vi "Make_Different_Variants_of_Tracks-6.vi"(8 "error IN":errorcluster, 9 "[IN] # of Longest track\nInside the Group of Tracks":i32, 10 "[IN] Index of Earliest \nProblem Point Inside":i32, 11 "[IN] Still connected\ntracks in group":T2) -> (0 "error OUT":errorcluster, 1 "[OUT] Index of # tracks \nwith problem points":i32[](array[numeric]), 2 "[OUT] Index of connected \npoints inside the track":i32[](array[numeric]), 3 "[OUT] Subtracks":T1(array[cluster]), 4 "[OUT] Status of 1st Problem Point":i16, 5 "[OUT] 2 or more subtracks":bool)   [LabVIEW 2017]
doc: "The subVI formates competing subtracks \nTwo cases are considered: \nSplitting event => only variants after splitting + account the origin of one of subtracks\nMerging event => competition between different variants of elongations"
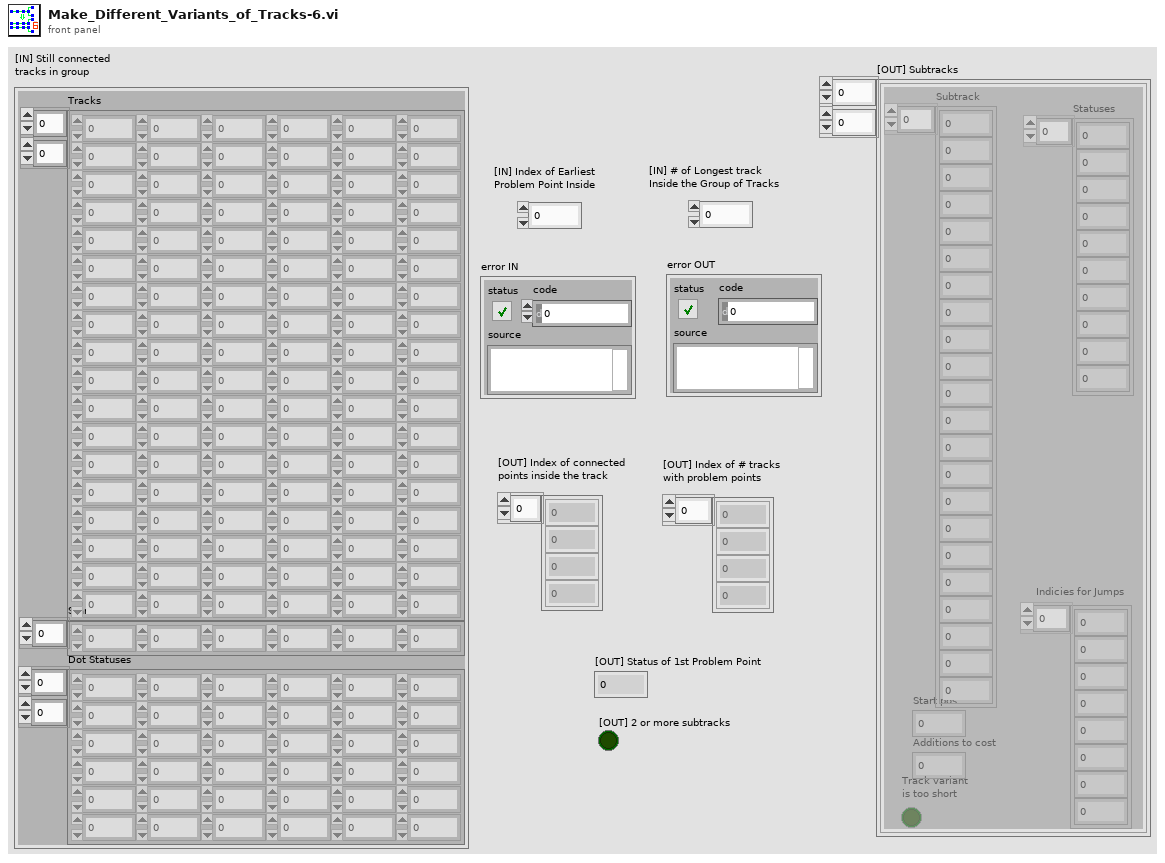
[diagram p1: front panel]
types:
  T1 = cluster{"Subtrack":dbl[], "Statuses":i16[], "Start pos":i32, "Additions to cost":i8, "Track variant \nis too short":bool, "Indicies for Jumps":i32[]}[][]
  T2 = cluster{"Tracks":dbl[][], "Start Pos":i32[], "Dot Statuses":i16[][]}
  T3 = cluster{"Subtrack":dbl[], "Statuses":i16[], "Start pos":i32, "Additions to cost":i8, "Track variant \nis too short":bool, "Indicies for Jumps":i32[]}
  T4 = cluster{"Subtrack":dbl[], "Statuses":i16[], "Start pos":i32, "Additions to cost":i8, "Track variant \nis too short":bool, "Indicies for Jumps":i32[]}[]
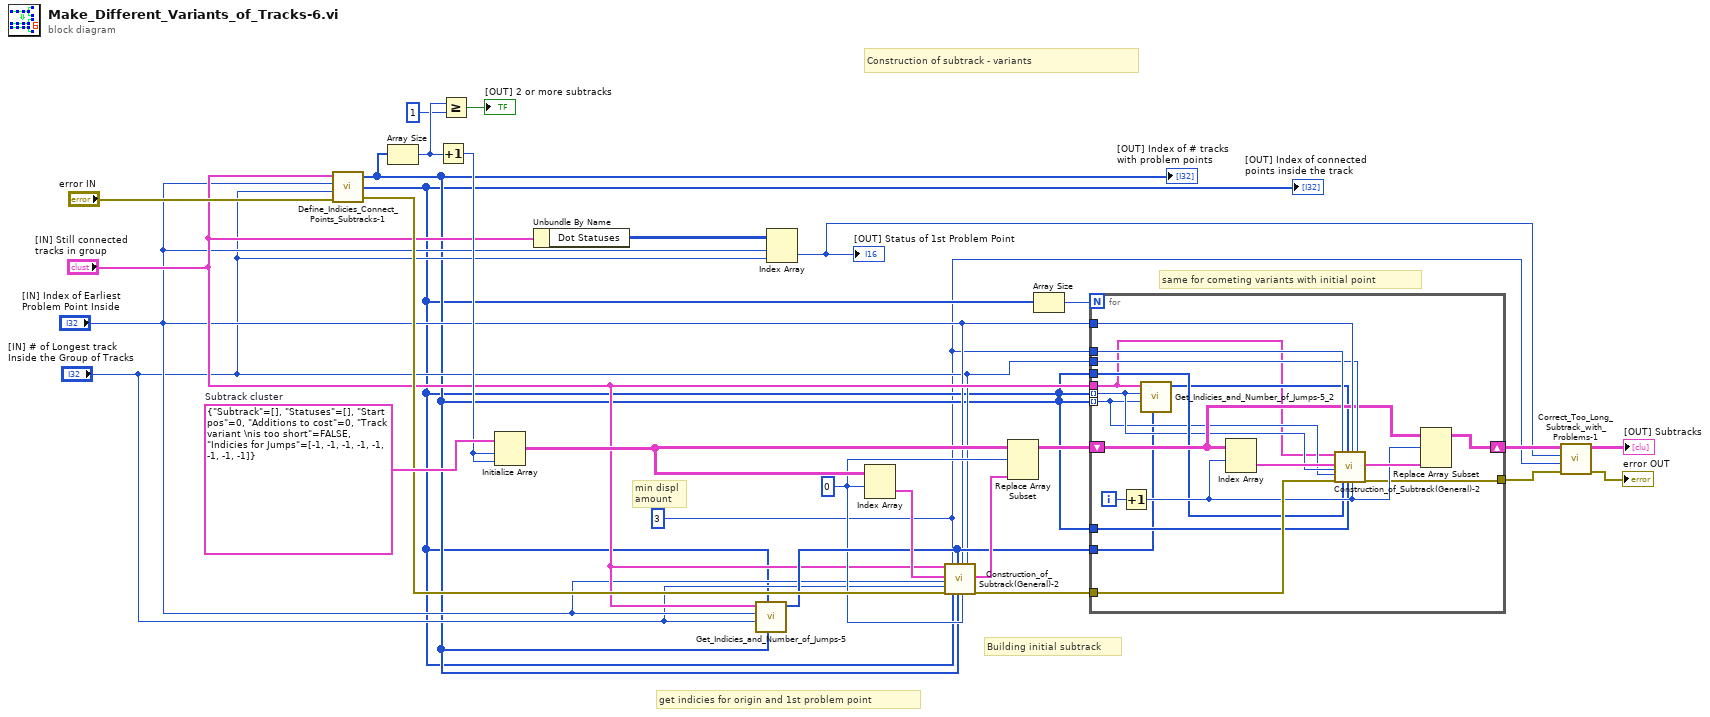
[diagram p0: block diagram]
diagram:
  w16 = 0
  w1 = 3 ("[IN] Minimal Subtrack Length \n(Points without problems) for\nMaking Desicion")
  w27 = T3 {"Subtrack"=[], "Statuses"=[], "Start pos"=0, "Additions to cost"=0, "Track variant \nis too short"=FALSE, "Indicies for Jumps"=[-1, -1, -1, -1, -1, -1, -1, -1]}  # Subtrack cluster
  # "same for cometing variants with initial point"
  # "Building initial subtrack"
  # "get indicies for origin and 1st problem point"
  # "min displ \namount"
  # "Construction of subtrack - variants"
  n1 = call "Define_Indicies_Connect_Points_Subtracks-1.vi"("error IN"="error IN", "[IN] Index of track with\n(problem displacement)"="[IN] # of Longest track\nInside the Group of Tracks", "[IN] Index of problem\ndisplacement inside track"="[IN] Index of Earliest \nProblem Point Inside", "[IN] Track group"="[IN] Still connected\ntracks in group") -> ("error OUT"=w18:errorcluster, "[OUT] Index of \nconnected dots\ninside the track"=w10:i32[], "[OUT] Index of connected\ntracks with problem dot"=w11:i32[])
  "[OUT] Index of connected \npoints inside the track" <- w10
  "[OUT] Index of # tracks \nwith problem points" <- w11
  n2 = Array Size(array=w11) -> (size(s)=w9:i32)
  n3 = Increment(x=w9) -> (x+1=w23:i32)
  n4 = Greater Or Equal?(x=w9, y=1) -> (x >= y?=→"[OUT] 2 or more subtracks":bool)
  n5 = Initialize Array(w27, w23, w23) -> (w26:T1)
  n6 = Unbundle By Name("[IN] Still connected\ntracks in group") -> ("Dot Statuses"=w14:i16[][])
  n7 = call "Get_Indicies_and_Number_of_Jumps-5.vi"("[IN] Index of connected\ntracks with problem dot"=w11, "[IN] Index of connected \ndots inside the track"=w10, "[IN] # of Track with\nFirst Problem Point"="[IN] # of Longest track\nInside the Group of Tracks", "[IN] Index of First Pro\nblem Point Inside Track"="[IN] Index of Earliest \nProblem Point Inside", "[IN] Still connected\ntracks in group"="[IN] Still connected\ntracks in group") -> ("[OUT] Indicies for Jumps"=w17:i32[])  [unwired: 5 in]
  n8 = Index Array(array=w14, index (row)="[IN] Index of Earliest \nProblem Point Inside", index (col)="[IN] # of Longest track\nInside the Group of Tracks") -> (element=w2:i16)
  "[OUT] Status of 1st Problem Point" <- w2
  n9 = Index Array(array=w26, index (row)=w16) -> (element=w19:T4)  [unwired: 1 in]
  n10 = call "Construction_of_Subtrack(General)-2.vi"("[IN] Still connected\ntracks in group"="[IN] Still connected\ntracks in group", "[IN] Subtrack (Row of variants)"=w19, "[IN] Index of First Pro\nblem Point Inside Track"="[IN] Index of Earliest \nProblem Point Inside", "[IN] # of Track with\nFirst Problem Point"="[IN] # of Longest track\nInside the Group of Tracks", "error IN"=w18, "[IN] Minimal Subtrack Len\ngth for Making Desicion"=w1, "[IN] Index of \nconnected dots\ninside the track"=w10, "[IN] Indexes for Jumps"=w17, "[IN] Index of connected\ntracks with problem dot"=w11, "[IN] Index of Initial Pro\nblem Point Inside Track"="[IN] Index of Earliest \nProblem Point Inside", "[IN] # of Problem Row"=w16, "[IN] # of Track with\ninitial Problem Point"="[IN] # of Longest track\nInside the Group of Tracks") -> ("[OUT] Subtracks"=w20:T4, "error OUT"=w21:errorcluster)  [unwired: 6 in]
  n11 = Replace Array Subset(array=w26, new element=w20, index (row)=w16) -> (w25:T1)  [unwired: 1 in]
  n12 = Array Size(array=w10) -> (size(s)=w24:i32)
  n13 = for {
    N: w24 -> [_]
    shift-right: [w37] -> w6
    shift-left: w25 -> [w39]
    tunnel: "[IN] Still connected\ntracks in group" -> [w28]
    tunnel: w21 -> [w40]
    tunnel: w10 -> [w32] mode=indexing
    tunnel: w11 -> [w31] mode=indexing
    tunnel: w1 -> [w43]
    tunnel: w17 -> [w29]
    tunnel: w10 -> [w34]
    tunnel: w11 -> [w35]
    tunnel: "[IN] # of Longest track\nInside the Group of Tracks" -> [w41]
    tunnel: "[IN] Index of Earliest \nProblem Point Inside" -> [w42]
    tunnel: [w33] -> w3
    i -> [w45]
    n14 = Increment(x=w45) -> (x+1=w36:i32)
    n15 = call "Get_Indicies_and_Number_of_Jumps-5_2.vi"("[IN] Indicies for Jumps"=w29, "[IN] # of Track with\nFirst Problem Point"=w31, "[IN] Index of First Pro\nblem Point Inside Track"=w32, "[IN] Still connected\ntracks in group"=w28) -> ("[OUT] Indexes for Jumps"=w30:i32[])  [unwired: 6 in]
    n16 = Index Array(array=w39, index (row)=w36) -> (element=w44:T4)  [unwired: 1 in]
    n17 = call "Construction_of_Subtrack(General)-2.vi"("[IN] Still connected\ntracks in group"=w28, "[IN] Subtrack (Row of variants)"=w44, "[IN] Index of First Pro\nblem Point Inside Track"=w32, "[IN] # of Track with\nFirst Problem Point"=w31, "error IN"=w40, "[IN] Minimal Subtrack Len\ngth for Making Desicion"=w43, "[IN] Index of \nconnected dots\ninside the track"=w34, "[IN] Indexes for Jumps"=w30, "[IN] Index of connected\ntracks with problem dot"=w35, "[IN] Index of Initial Pro\nblem Point Inside Track"=w42, "[IN] # of Problem Row"=w36, "[IN] # of Track with\ninitial Problem Point"=w41) -> ("[OUT] Subtracks"=w38:T4, "error OUT"=w33:errorcluster)  [unwired: 6 in]
    n18 = Replace Array Subset(array=w39, new element=w38, index (row)=w36) -> (w37:T1)  [unwired: 1 in]
  }
  n19 = call "Correct_Too_Long_Subtrack_with_Problems-1.vi"("error IN"=w3, "[IN] Minimal Subtrack Len\ngth for Making Desicion"=w1, "[IN] Status of problem point"=w2, "[IN] Subtracks"=w6) -> ("error OUT"=→"error OUT":errorcluster, "[OUT] Subtracks"=→"[OUT] Subtracks":T1)  [unwired: 2 in]
